vi "Stepper Change Direction.vi"(2 "Wait before changing (Ticks)":u8=3, 3 "Direction (T=Home)":bool) -> ()   [LabVIEW 2015]
uses:
  <vilib>/rvi/eio/common/nirviEmuTemplateMethod_errors.vi
  <vilib>/eio/EIONode/EIONode.xnode
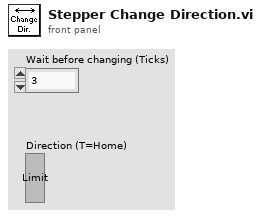
[diagram p1: front panel]
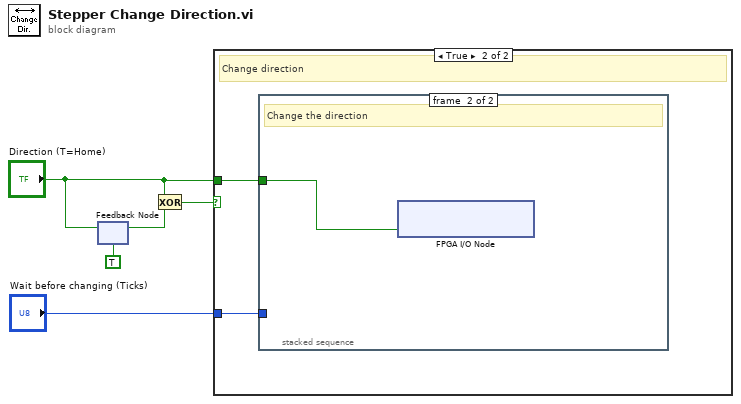
[diagram p0: block diagram]
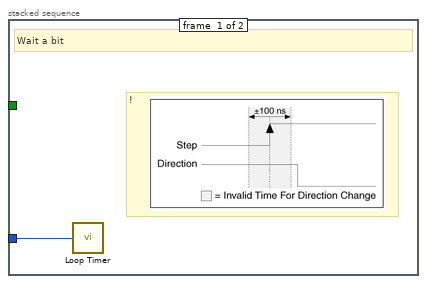
[diagram p3: hidden frame]
diagram:
  n1 = feedback #1(TRUE) -> (w4:bool)
  n2 = feedback-in #1("Direction (T=Home)") -> ()
  n3 = Exclusive Or(1:w4, 2:"Direction (T=Home)") -> (0:w3:bool)
  n4 = case shown="True" w3 {
    tunnel: "Direction (T=Home)" -> [_ w6]
    tunnel: "Wait before changing (Ticks)" -> [_ w7]
    frame False {
    }
    frame True {
      # "Change direction"
      n5 = stacked-sequence {
        tunnel: w7 -> [w8 _]
        tunnel: w6 -> [_ w9]
        frame #0 {
          # "!"
          # "Wait a bit"
          n6 = call "Loop Timer"("Count(Ticks)"=w8) -> ()  [unwired: 1 out]
        }
        frame #1 {
          # "Change the direction"
          n7 = xnode "FPGA I/O Node"("Stepper/Direction"=w9) -> ()  [unwired: 1 in, 1 out]
        }
      }
    }
  }
